vi "Read Variable (string).vi"(8 "error in (no error)":errorcluster, 9 "Datatype":string, 10 "PG path":string, 11 "Data.PGQL in":refnum<class "LV-Data.PGSQL.lvclass">) -> (0 "error out":errorcluster, 1 "Time Stamp":timestamp, 2 "Value":string, 3 "Data.PGSQL out":refnum<class "LV-Data.PGSQL.lvclass">, 4 "Column (units)":string, 5 "SQL string":string)   [LabVIEW 2019, in "LV-Data.PGSQL.lvclass"]
uses:
  LV-Data.PGSQL.lvclass
  <vilib>/JDP Science/PostgreSQL Library/Connection/PQ Connection.lvclass
  LV-Data.PGSQL.lvclass/LV-Data.PGSQL.ctl
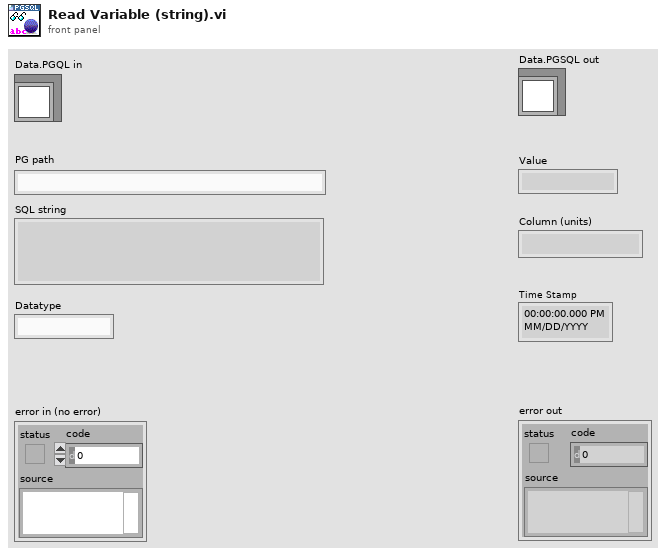
[diagram p1: front panel]
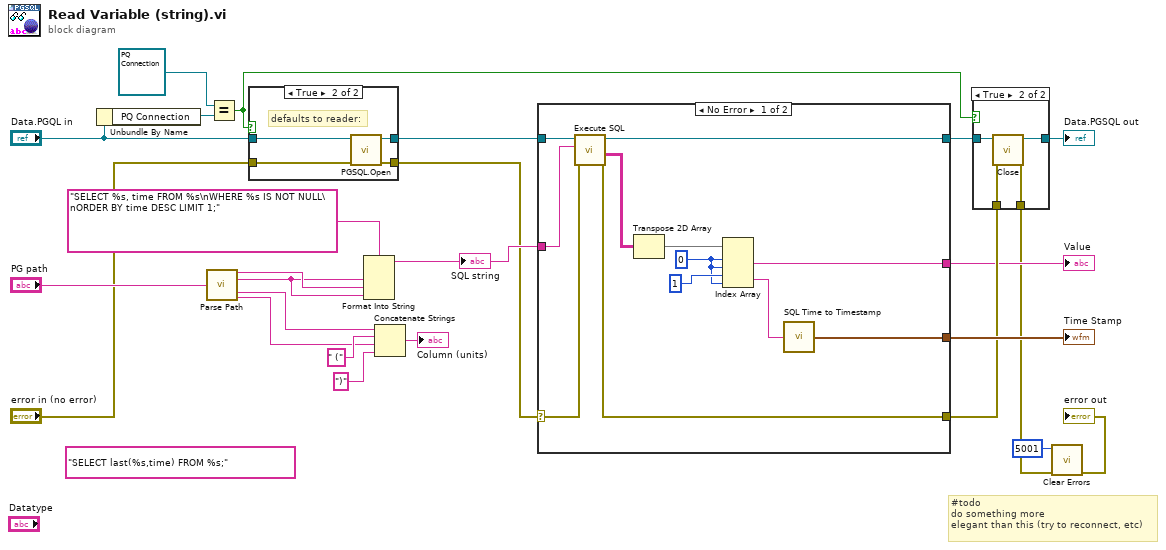
[diagram p0: block diagram]
diagram:
  (unwired) "SELECT last(%s,time) FROM %s;" ("format string")
  # "#todo\ndo something more\nelegant than this (try to reconnect, etc)"
  n1 = Unbundle By Name("Data.PGQL in") -> ("PQ Connection"=w4:refnum<class "PQ Connection.lvclass">)
  n2 = call "Parse Path.vi"("PG Path"="PG path") -> ("Table path"=w22:string, "Column path"=w8:string, "Column name"=w18:string, "Column units"=w19:string)  [unwired: 10 in, 1 out]
  n3 = Equal?(x=refnum<class "PQ Connection.lvclass"> refnum ("PQ Connection"), y=w4) -> (x = y?=w1:bool)
  n4 = case shown="True" w1 {
    tunnel: "Data.PGQL in" -> [w27 w29]
    tunnel: "error in (no error)" -> [w26 w28]
    tunnel: [w27 w31] -> w15
    tunnel: [w26 w30] -> w14
    frame False {
    }
    frame True {
      # "defaults to reader:"
      n5 = call "PGSQL.Open.vi"("error in (no error)"=w28, "Data.PG in"=w29) -> ("error out"=w30:errorcluster, "Data.PG out"=w31:refnum<class "LV-Data.PGSQL.lvclass">)  [unwired: 8 in]
    }
  }
  n6 = Format Into String(format string="SELECT %s, time FROM %s\nWHERE %s IS NOT NULL\nORDER BY time DESC LIMIT 1;", w8, w22, w8) -> (resulting string=w20:string)  [unwired: 2 in, 1 out]
  "SQL string" <- w20
  n7 = Concatenate Strings(w18, " (" ("string"), w19, ")" ("string")) -> (→"Column (units)":string)
  n8 = case shown="No Error" w14 {
    selector: w14 -> [w38 w44]
    tunnel: w15 -> [w42 w45]
    tunnel: w20 -> [w39 _]
    tunnel: [w41 w44] -> w11
    tunnel: [w40 w45] -> w13
    tunnel: [w33 _] -> w9
    tunnel: [w36 _] -> w17
    frame No Error {
      w34 = 0 ("index (row)")
      n9 = call "Execute SQL.vi"("error in"=w38, "SQL"=w39, "LV-Data.PGSQL"=w42) -> ("error out"=w41:errorcluster, "Result"=w32:string[][], "LV-Data.PGSQL out"=w40:refnum<class "LV-Data.PGSQL.lvclass">)  [unwired: 5 in, 1 out]
      n10 = Transpose 2D Array(2D array=w32) -> (transposed array=w43:string[][])
      n11 = Index Array(array=w43, index (row) #1=w34, index (col) #1=w34, index (row) #2=1 ("index (row)"), index (col) #2=w34) -> (element #1=w33:string, element #2=w37:string)
      n12 = call "SQL Time to Timestamp.vi"("date/time string"=w37) -> ("Time Stamp"=w36:timestamp)
    }
    frame Error {
    }
  }
  "Time Stamp" <- w17
  "Value" <- w9
  n13 = case shown="True" w1 {
    tunnel: w13 -> [w47 w51]
    tunnel: [w47 w50] -> w12
    tunnel: w11 -> [w46 w49]
    tunnel: [w46 w48] -> w6
    frame False {
    }
    frame True {
      n14 = call-dynamic "Close.vi"("error in (no error)"=w49, "Data.PG in"=w51) -> ("error out"=w48:errorcluster, "Data.PG out"=w50:refnum<class "LV-Data.PGSQL.lvclass">)  [unwired: 8 in]
    }
  }
  "Data.PGSQL out" <- w12
  n15 = call <vilib>:"Clear Errors.vi"("error in (no error)"=w6, "specific error code to clear (0: all)"=5001) -> ("error out"=→"error out":errorcluster)  [unwired: 4 in, 1 out]
